vi "Periodic Tasks.vi"() -> ()   [LabVIEW 2011]
doc: "This VI runs in parallel to other tasks. It can contain as many user-defined periodic loops as you need. These can carry out PID or other sorts of timed response."
uses:
  <vilib>/Rock Robotics/SystemInterfaces/Utilities/FPGA_UtilitiesLED State.ctl
  <vilib>/Rock Robotics/SystemInterfaces/Utilities/FPGA_UtilitiesLED Source.ctl
  <vilib>/Rock Robotics/WPI/Relay/WPI_RelayValue.ctl
  Robot Global Data.vi
panel:
  out "Heading 2":u16
  out "Angular Rate":dbl
  out "Angle":dbl
  out "Direction":bool
  out "Distance":dbl
  in  "Home Speed":dbl=1.0
  in  "Home Position":dbl=2.85
  out "Current Voltage":dbl
  in  "upper limit":dbl=4.5
  in  "lower limit":dbl=0.85
  # "Speed to move to home"
  # "Target Tracking"
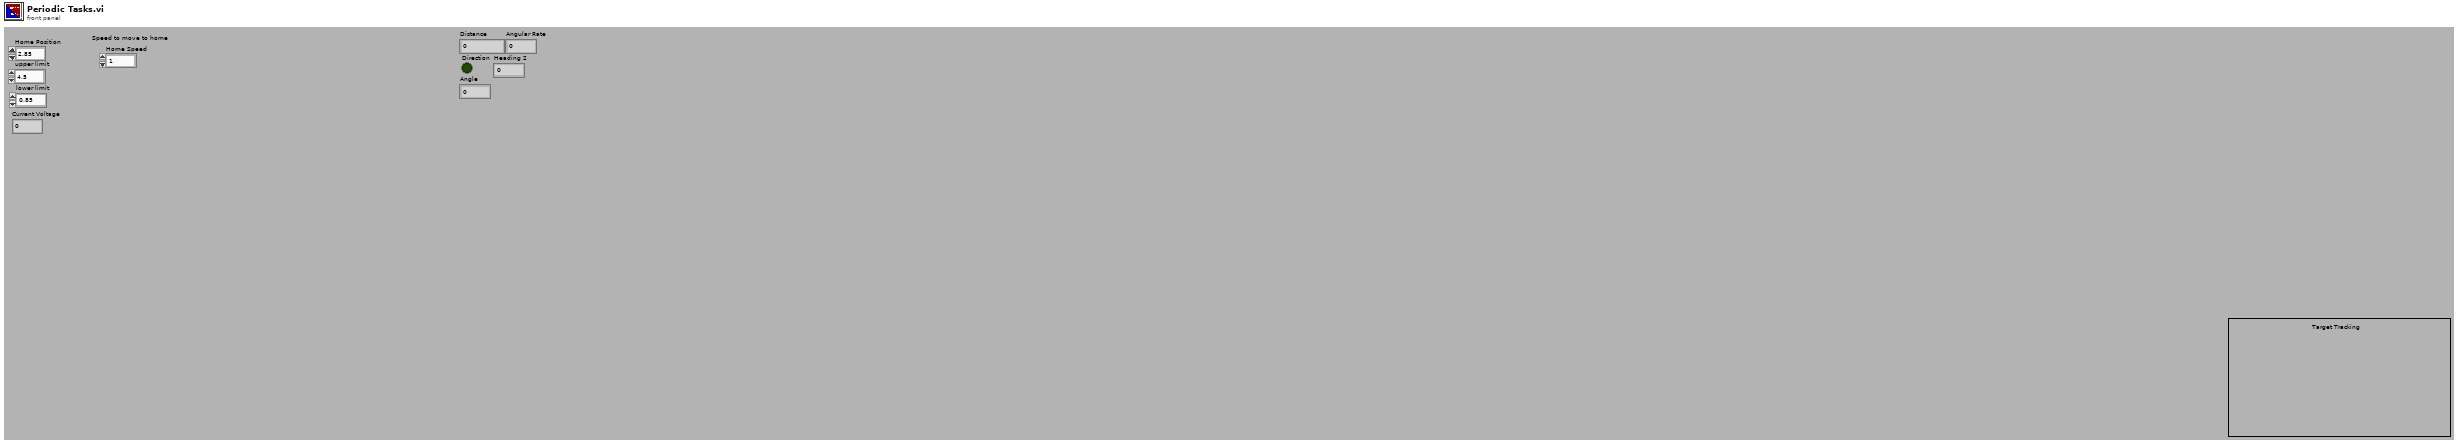
[diagram p1: front panel]
types:
  T1 = typedef "WPI_RelayValue.ctl" = enum16{"Off", "On", "Forward", "Reverse"}
  T2 = typedef "WPI_GyroDevRef.ctl" = cluster{"DevStatus":errorcluster, "Analog Module":T3, "Analog Channel":T4, "Offset":dbl, "Gain (VoltsPerDegree/Second)":dbl}
  T3 = typedef "FPGA_TypedefAnalogModule.ctl" = enum16{"Analog Module 1", "Analog Module 2"}
  T4 = typedef "FPGA_AIChannel.ctl" = enum8{"AI 1", "AI 2", "AI 3", "AI 4", "AI 5", "AI 6", "AI 7", "AI 8", "Invalid"}
  T5 = typedef "WPI_EncoderDevRef.ctl" = cluster{"DevStatus":errorcluster, "EncoderIndex":T6, "CounterIndex":T7, "DistancePerCount":dbl, "Decoding Type":T8}
  T6 = typedef "FPGA_EncoderIdx.ctl" = enum8{"Enc 0", "Enc 1", "Enc 2", "Enc 3", "Invalid"}
  T7 = typedef "FPGA_CounterCtrSystemIndex.ctl" = enum8{"Ctr 0", "Ctr 1", "Ctr 2", "Ctr 3", "Ctr 4", "Ctr 5", "Ctr 6", "Ctr 7", "Invalid"}
  T8 = typedef "WPI_EncoderType.ctl" = enum16{"1x", "2x", "4x"}
  T9 = typedef "WPI_AnalogChannelDevRef.ctl" = cluster{"DevStatus":errorcluster, "Analog Module":T3, "Analog Channel":T4}
  T10 = typedef "WPI_I2CDevRef.ctl" = cluster{"DevStatus":errorcluster, "Digital Module":T11, "Device Address":u8}
  T11 = typedef "FPGA_TypedefDigitalModule.ctl" = enum16{"Digital Module 1", "Digital Module 2"}
  T12 = typedef "WPI_RelayDevRef.ctl" = cluster{"DevStatus":errorcluster, "Relay Channel":T13, "Digital Module":T11, "Relay Direction":T14}
  T13 = typedef "FPGA_DIORelayChannel.ctl" = enum8{"Relay 1", "Relay 2", "Relay 3", "Relay 4", "Relay 5", "Relay 6", "Relay 7", "Relay 8", "Invalid"}
  T14 = typedef "WPI_RelayDirection.ctl" = enum16{"Both directions", "Forward only", "Reverse only"}
  T15 = cluster{"Driver Station Digital Output (1-8)[0]":bool, "Driver Station Digital Output (1-8)[1]":bool, "Driver Station Digital Output (1-8)[2]":bool, "Driver Station Digital Output (1-8)[3]":bool, "Driver Station Digital Output (1-8)[4]":bool, "Driver Station Digital Output (1-8)[5]":bool, "Driver Station Digital Output (1-8)[6]":bool, "Driver Station Digital Output (1-8)[7]":bool, "Driver Station Digital Output (1-8)[8]":bool}
  T16 = typedef "FPGA_UtilitiesLED State.ctl" = enum16{"Off", "On", "Toggle"}
  T17 = typedef "FPGA_UtilitiesLED Source.ctl" = enum16{"User LED", "FPGA LED"}
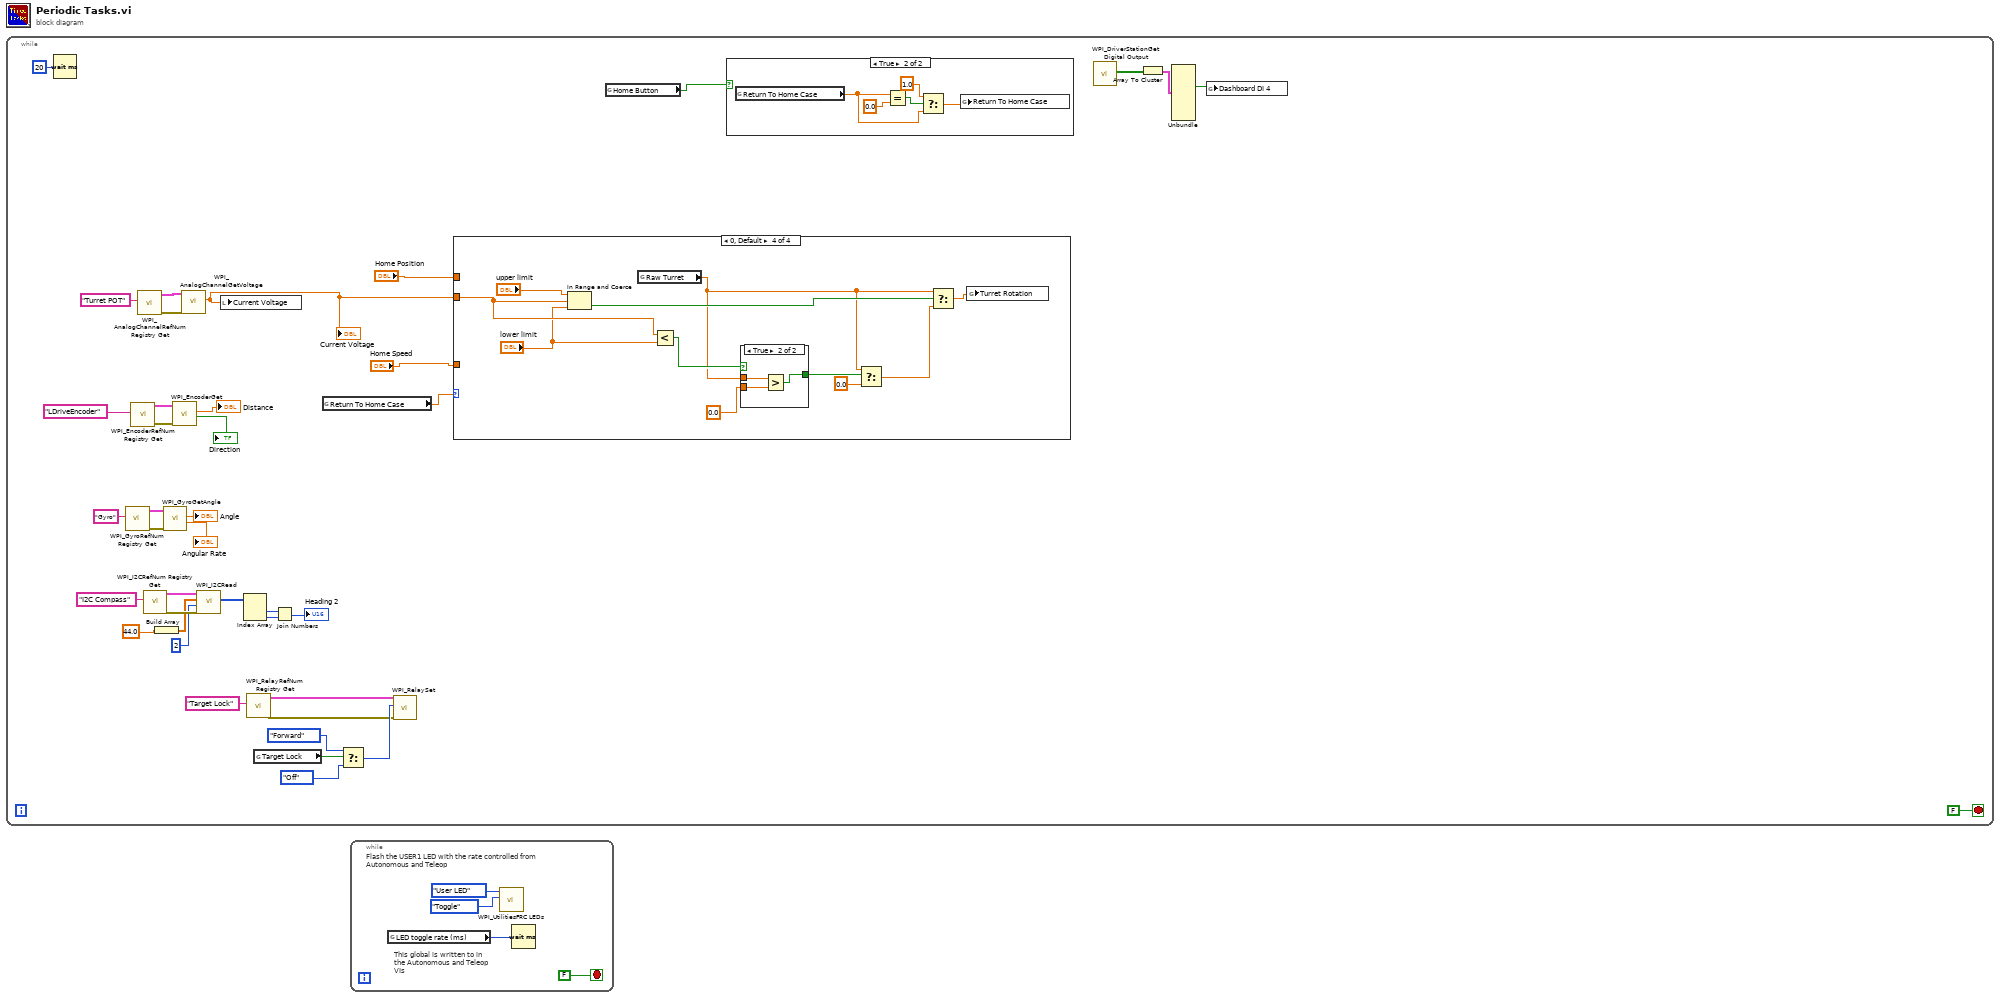
[diagram p0: block diagram]
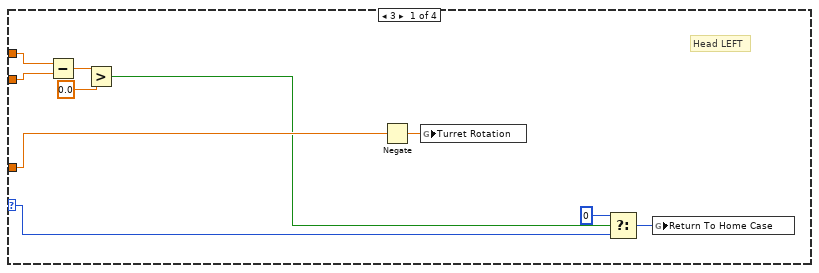
[diagram p2: hidden frame]
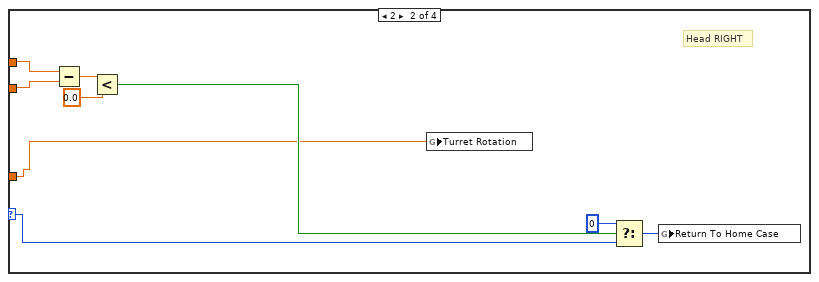
[diagram p3: hidden frame]
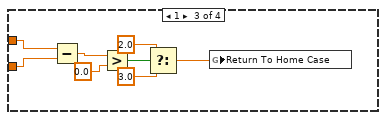
[diagram p4: hidden frame]
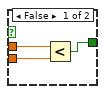
[diagram p5: hidden frame]
diagram:
  n1 = while {
    stop <- FALSE stop-if-true
    n2 = Wait (ms)(milliseconds to wait=u32 20) -> ()  [unwired: 1 out]
    n3 = call <vilib>:"WPI_GyroRefNum Registry Get.vi"("refnum name"="Gyro") -> ("error out"=w14:errorcluster, "GyroDevRef"=w15:T2)  [unwired: 9 in]
    n4 = call <vilib>:"WPI_EncoderRefNum Registry Get.vi"("refnum name"="LDriveEncoder") -> ("error out"=w17:errorcluster, "EncoderDevRef"=w18:T5)  [unwired: 9 in]
    n5 = call <vilib>:"WPI_AnalogChannelRefNum Registry Get.vi"("refnum name"="Turret POT") -> ("error out"=w20:errorcluster, "AIDeviceRef"=w21:T9)  [unwired: 9 in]
    n6 = call <vilib>:"WPI_I2CRefNum Registry Get.vi"("refnum name"="I2C Compass") -> ("error out"=w10:errorcluster, "I2CDevRef"=w9:T10)  [unwired: 9 in]
    n7 = Build Array(44.0 ("element")) -> (w3:dbl[])
    n8 = call <vilib>:"WPI_GyroGetAngle.vi"("error in (no error)"=w14, "GyroDevRef"=w15) -> ("Angular Rate"=→"Angular Rate":dbl, "Angle"=→"Angle":dbl)  [unwired: 6 in, 2 out]
    n9 = call <vilib>:"WPI_EncoderGet.vi"("error in (no error)"=w17, "EncoderDevRef"=w18) -> ("Direction"=→"Direction":bool, "Distance"=→"Distance":dbl)  [unwired: 4 in, 4 out]
    n10 = call <vilib>:"WPI_AnalogChannelGetVoltage.vi"("error in (no error)"=w20, "AIDeviceRef"=w21) -> ("Voltage"=w29:dbl)  [unwired: 7 in, 2 out]
    "Current Voltage" <- w29
    n11 = call <vilib>:"WPI_I2CRead.vi"("error in (no error)"=w10, "I2CBytesToRead"=u8 2, "I2CRegister"=w3, "I2CDevRef"=w9) -> ("Data Out"=w7:u8[])  [unwired: 5 in, 2 out]
    n12 = local write "Current Voltage"(w29) -> ()
    n13 = Index Array(array=w7) -> (element #1=w5:u8, element #2=w6:u8)  [unwired: 2 in]
    n14 = call <vilib>:"WPI_RelayRefNum Registry Get.vi"("refnum name"="Target Lock") -> ("error out"=w31:errorcluster, "RelayDevRef"=w32:T12)  [unwired: 9 in]
    n15 = global read "Robot Global Data.vi" "Target Lock"() -> (w37:bool)
    n16 = Join Numbers(hi=w5, lo=w6) -> ((hi.lo)=→"Heading 2":u16)
    n17 = global read "Robot Global Data.vi" "Return To Home Case"() -> (w28:dbl)
    n18 = Select(t=WPI_RelayValue."Forward" ("RelayValue"), s=w37, f=WPI_RelayValue."Off" ("RelayValue")) -> (s? t:f=w34:T1)
    n19 = call <vilib>:"WPI_RelaySet.vi"("error in (no error)"=w31, "RelayValue"=w34, "RelayDevRef"=w32) -> ()  [unwired: 7 in, 2 out]
    n20 = case shown="0, Default" w28 {
      selector: w28 -> [w48 w52 _ _]
      tunnel: w29 -> [w44 w53 w66 w78]
      tunnel: "Home Position" -> [w45 w54 w67 _]
      tunnel: "Home Speed" -> [w46 w51 _ _]
      frame 3 {
        # "Head LEFT"
        n21 = Subtract(x=w45, y=w44) -> (x-y=w43:dbl)
        n22 = Greater?(x=w43, y=0.0) -> (0:w41:bool)
        n23 = Negate(x=w46) -> (-x=w47:dbl)
        n24 = global write "Robot Global Data.vi" "Turret Rotation"(w47) -> ()
        n25 = Select(t=0, s=w41, f=w48) -> (s? t:f=w49:i32)
        n26 = global write "Robot Global Data.vi" "Return To Home Case"(w49) -> ()
      }
      frame 2 {
        # "Head RIGHT"
        n27 = Subtract(x=w54, y=w53) -> (x-y=w57:dbl)
        n28 = Less?(x=w57, y=0.0) -> (x < y?=w55:bool)
        n29 = global write "Robot Global Data.vi" "Turret Rotation"(w51) -> ()
        n30 = Select(t=0, s=w55, f=w52) -> (s? t:f=w58:i32)
        n31 = global write "Robot Global Data.vi" "Return To Home Case"(w58) -> ()
      }
      frame 1 {
        n32 = Subtract(x=w67, y=w66) -> (x-y=w65:dbl)
        n33 = Greater?(x=w65, y=0.0) -> (0:w63:bool)
        n34 = Select(t=2.0, s=w63, f=3.0) -> (s? t:f=w60:dbl)
        n35 = global write "Robot Global Data.vi" "Return To Home Case"(w60) -> ()
      }
      frame 0, Default {
        n36 = In Range and Coerce(upper limit="upper limit", x=w78, lower limit="lower limit") -> (In Range?=w75:bool)  [unwired: 1 out]
        n37 = global read "Robot Global Data.vi" "Raw Turret"() -> (w68:dbl)
        n38 = Less?(x=w78, y="lower limit") -> (x < y?=w70:bool)
        n39 = case shown="True" w70 {
          tunnel: 0.0 -> [w80 w84]
          tunnel: [w79 w83] -> w71
          tunnel: w68 -> [w81 w82]
          frame False {
            n40 = Less?(x=w81, y=w80) -> (x < y?=w79:bool)
          }
          frame True {
            n41 = Greater?(x=w82, y=w84) -> (0:w83:bool)
          }
        }
        n42 = Select(t=w68, s=w71, f=0.0) -> (s? t:f=w69:dbl)
        n43 = Select(t=w68, s=w75, f=w69) -> (s? t:f=w77:dbl)
        n44 = global write "Robot Global Data.vi" "Turret Rotation"(w77) -> ()
      }
    }
    n45 = global read "Robot Global Data.vi" "Home Button"() -> (w25:bool)
    n46 = case shown="True" w25 {
      frame False {
      }
      frame True {
        n47 = global read "Robot Global Data.vi" "Return To Home Case"() -> (w86:dbl)
        n48 = Equal?(x=w86, y=0.0) -> (x = y?=w88:bool)
        n49 = Select(t=1.0, s=w88, f=w86) -> (s? t:f=w85:dbl)
        n50 = global write "Robot Global Data.vi" "Return To Home Case"(w85) -> ()
      }
    }
    n51 = call <vilib>:"WPI_DriverStationGet Digital Output.vi"() -> ("Driver Station Digital Output (1-8)"=w40:bool[])  [unwired: 10 in, 1 out]
    n52 = Array To Cluster(array=w40) -> (cluster=w39:T15)
    n53 = Unbundle(w39) -> ("Driver Station Digital Output (1-8)[3]"=w38:bool)  [unwired: 8 out]
    n54 = global write "Robot Global Data.vi" "Dashboard DI 4"(w38) -> ()
  }
  n55 = while {
    stop <- FALSE stop-if-true
    # "This global is written to in the Autonomous and Teleop VIs"
    # "Flash the USER1 LED with the rate controlled from Autonomous and Teleop"
    n56 = global read "Robot Global Data.vi" "LED toggle rate (ms)"() -> (w90:u32)
    n57 = call <vilib>:"WPI_UtilitiesFRC LEDs.vi"("State"=FPGA_UtilitiesLED_State."Toggle", "LED Type"=FPGA_UtilitiesLED_Source."User LED") -> ()  [unwired: 1 in, 9 out]
    n58 = Wait (ms)(milliseconds to wait=w90) -> ()  [unwired: 1 out]
  }
